vi "Configure Math Operation.vi"(0 "VISA resource name":refnum<visa-resource-name>, 1 "Function":u16(ring) items=["Voltage: DC", "Voltage: AC", "Current: DC", "Current: AC", "2W Resistance", "4W Resistance", "Diode", "Capacitance", "Temperature", "Continuity", "Frequency", "Period", "Ratio", "Digitize Voltage", "Digitize Current"], 2 "Math Operation (1: Percent)":u16(ring)=1 items=["Y= mx+b", "Percent", "Reciprocal"], 3 "M Value (1)":dbl=1.0, 4 "B Value (0)":dbl, 5 "error in (no error)":errorcluster, 7 "Percent Value (1)":dbl=1.0) -> (14 "VISA resource name out":refnum<visa-resource-name>, 19 "error out":errorcluster)   [LabVIEW 2016, in "Keithley DMM7510.lvlib"]
doc: "This VI configures which math operation is performed on measurements. It also configures the related parameters like M,B value and percent etc.\nThe math operations:\n• y = mx+b\n• Percent\n• Reciprocal"
uses:
  Keithley DMM7510.lvlib
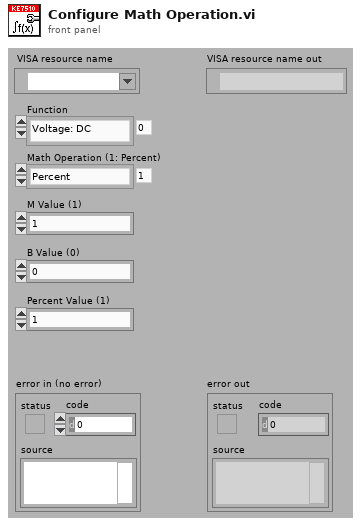
[diagram p1: front panel]
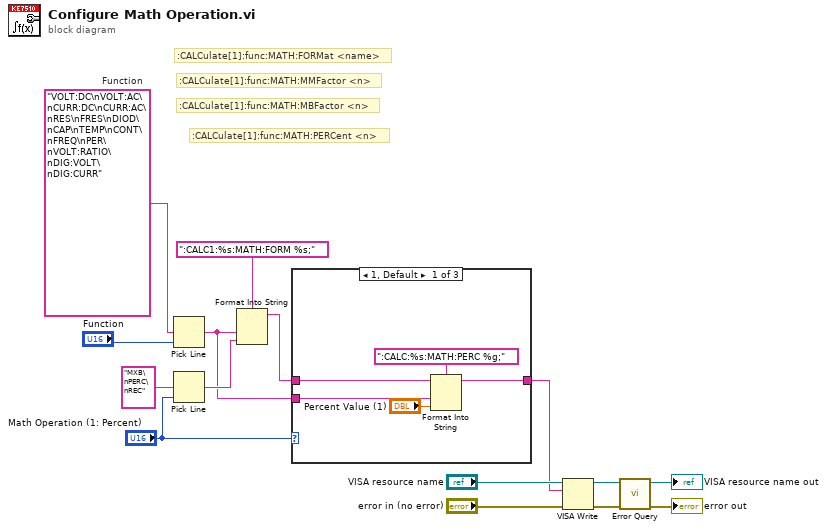
[diagram p0: block diagram]
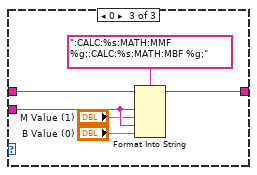
[diagram p3: hidden frame]
diagram:
  w1 = "VOLT:DC\nVOLT:AC\nCURR:DC\nCURR:AC\nRES\nFRES\nDIOD\nCAP\nTEMP\nCONT\nFREQ\nPER\nVOLT:RATIO\nDIG:VOLT\nDIG:CURR"  # Function
  # ":CALCulate[1]:func:MATH:FORMat <name>"
  # ":CALCulate[1]:func:MATH:MBFactor <n>"
  # ":CALCulate[1]:func:MATH:MMFactor <n>"
  # ":CALCulate[1]:func:MATH:PERCent <n>"
  n1 = Pick Line(multi-line string=w1, line index="Function") -> (output string=w6:string)  [unwired: 1 out]
  n2 = Pick Line(multi-line string="MXB\nPERC\nREC", line index="Math Operation (1: Percent)") -> (output string=w8:string)  [unwired: 1 out]
  n3 = Format Into String(format string=":CALC1:%s:MATH:FORM %s;", w6, w8) -> (resulting string=w5:string)  [unwired: 2 in, 1 out]
  n4 = case shown="1, Default" "Math Operation (1: Percent)" {
    tunnel: w6 -> [w19 _ w26]
    tunnel: w5 -> [w17 w21 w23]
    tunnel: [w16 w21 w22] -> w4
    frame 1, Default {
      n5 = Format Into String(format string=":CALC:%s:MATH:PERC %g;", initial string=w17, w19, "Percent Value (1)") -> (resulting string=w16:string)  [unwired: 1 in, 1 out]
    }
    frame 2 {
    }
    frame 0 {
      n6 = Format Into String(format string=":CALC:%s:MATH:MMF %g;:CALC:%s:MATH:MBF %g;", initial string=w23, w26, "M Value (1)", w26, "B Value (0)") -> (resulting string=w22:string)  [unwired: 1 in, 1 out]
    }
  }
  n7 = VISA Write(VISA resource name="VISA resource name", write buffer=w4, error in (no error)="error in (no error)") -> (VISA resource name out=w13:refnum<visa-resource-name>, error out=w10:errorcluster)  [unwired: 1 out]
  n8 = call "Error Query.vi"("error in (no error)"=w10, "VISA resource name"=w13) -> ("error out"=→"error out":errorcluster, "VISA resource name out"=→"VISA resource name out":refnum<visa-resource-name>)  [unwired: 6 in, 2 out]
